vi "T.vi"(8 "error in (no error)":errorcluster, 10 "Wire in":T1, 11 "Gate in":refnum<class "G-UE.lvclass">) -> (0 "error out":errorcluster, 3 "Gate out":refnum<class "G-UE.lvclass">)   [LabVIEW 2016, in "G-UE.lvclass"]
uses:
  G-UE.lvclass
  TypeDefs/Circuit Cluster.ctl
  GateAbst/GateAbst.lvclass
  <vilib>/Analysis/Matrix/Datatypes/ComplexMatrix.ctl
  <vilib>/Analysis/Matrix/NI_Matrix.lvlib
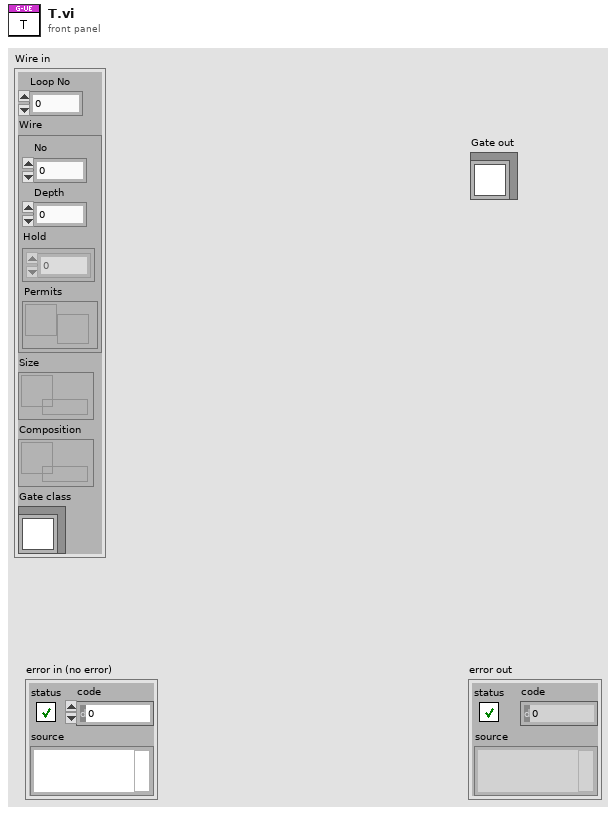
[diagram p1: front panel]
types:
  T1 = typedef "Circuit Cluster.ctl" = cluster{"Loop No":i32, "Wire":cluster{"No":i32, "Depth":i32, "Hold":i32[][], "Permits":refnum<notifier>}, "Size":refnum<queue>, "Composition":refnum<queue>, "Gate class":refnum<class "GateAbst.lvclass">}
  T2 = typedef "NI_Matrix.lvlib/ComplexMatrix.ctl" = cdb[][]
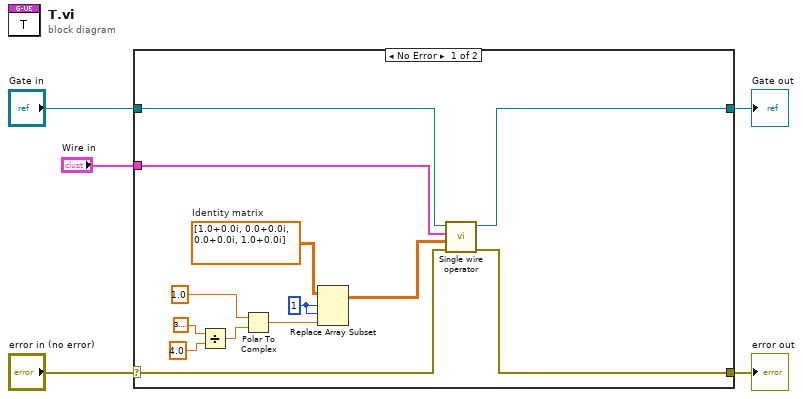
[diagram p0: block diagram]
diagram:
  n1 = case shown="No Error" "error in (no error)" {
    selector: "error in (no error)" -> [w15 w20]
    tunnel: [w16 w20] -> w4
    tunnel: [w17 w19] -> w2
    tunnel: "Gate in" -> [w18 w19]
    tunnel: "Wire in" -> [w6 _]
    frame No Error {
      w13 = 1 ("disabled index (row)")
      w14 = T2 [[1.0+0.0i, 0.0+0.0i], [0.0+0.0i, 1.0+0.0i]]  # Identity matrix
      n2 = Divide(x=3.141592653589793 ("Pi"), y=4.0) -> (x/y=w9:dbl)
      n3 = Polar To Complex(1:w9, 2:1.0 ("r")) -> (0:w11:cdb)
      n4 = Replace Array Subset ("Set Matrix Elements")(array=w14, new element=w11, index (row)=w13, index (col)=w13) -> (w12:T2)
      n5 = call "Single wire operator.vi"("error in (no error)"=w15, "Operator matrix"=w12, "Wire in"=w6, "G-UE in"=w18) -> ("error out"=w16:errorcluster, "G-UE out"=w17:refnum<class "G-UE.lvclass">)  [unwired: 6 in]
    }
    frame Error {
    }
  }
  "error out" <- w4
  "Gate out" <- w2
